vi "butterworth_waveform_filter.vi"(2 "high cutoff freq":dbl=10.0 format="%#_13g", 3 "low cutoff freq":dbl=0.05 format="%#_13g", 4 "input":waveform(dbl)(graph)) -> (1 "filtered":waveform(dbl)(graph))   [LabVIEW 2017]
uses:
  <vilib>/Analysis/3filter.llb/Filter Passband Type.ctl
  <vilib>/Analysis/3filter.llb/Butterworth Filter (DBL).vi
  <vilib>/Analysis/NI_AALBase.lvlib
panel:
  in  "order":i32=5
  out "original":waveform(dbl)(graph)
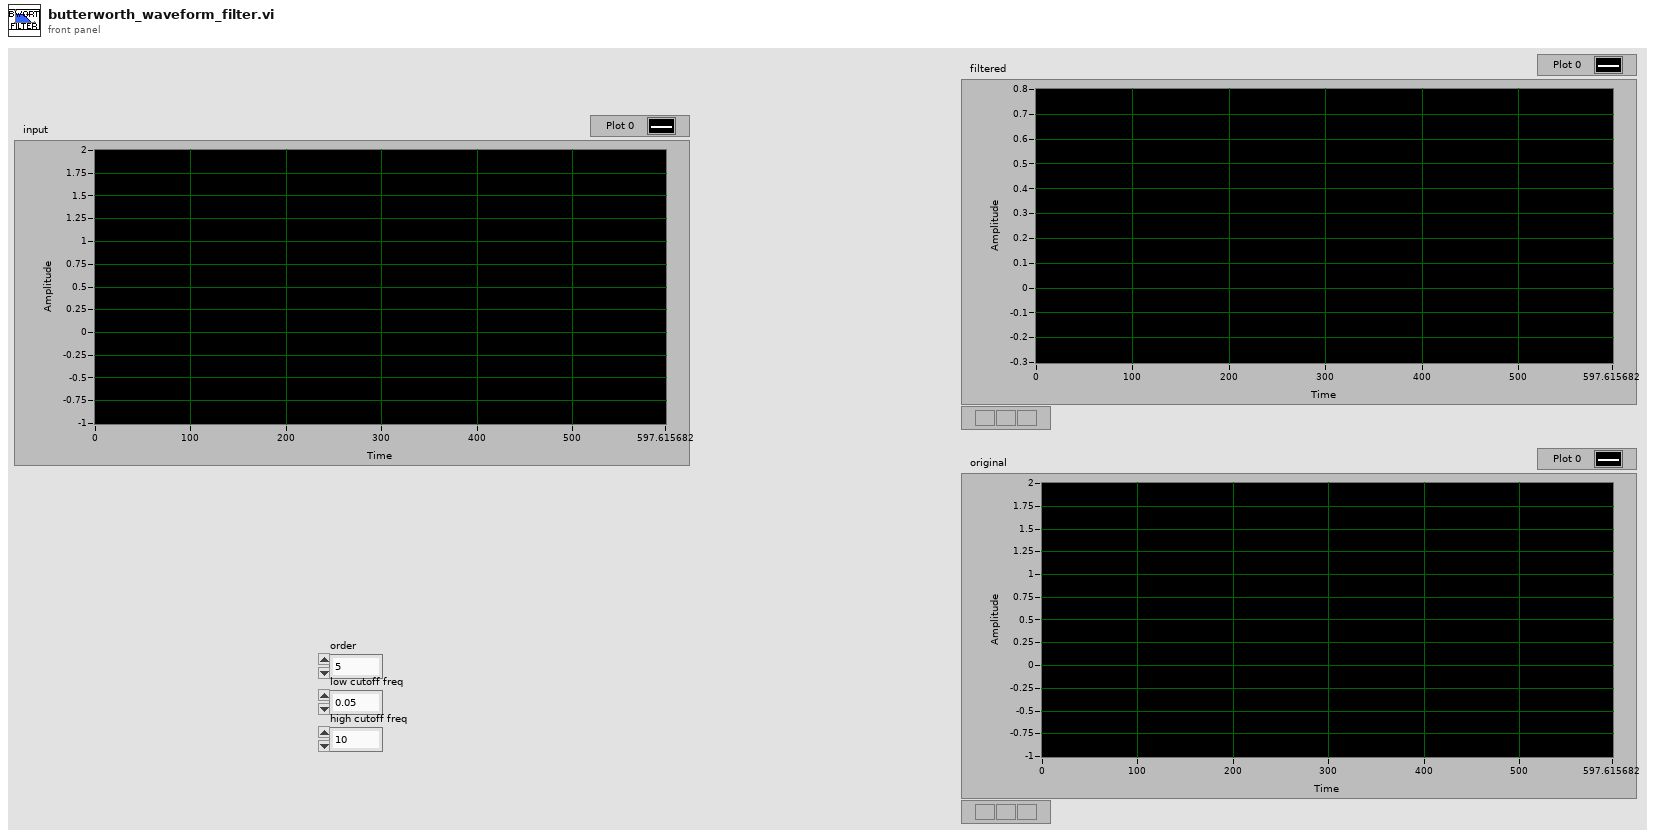
[diagram p1: front panel]
types:
  T1 = typedef "NI_AALBase.lvlib/Filter Passband Type.ctl" = enum32{"Lowpass", "Highpass", "Bandpass", "Bandstop"}
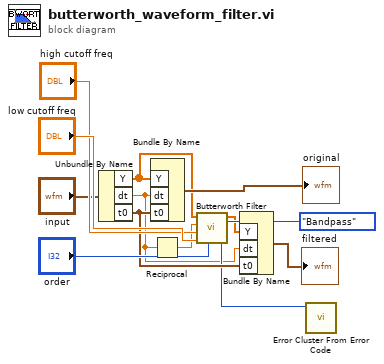
[diagram p0: block diagram]
diagram:
  n1 = Unbundle By Name("input") -> ("Y"=w6:dbl[], "dt"=w2:dbl, "t0"=w5:timestamp)
  n2 = Bundle By Name("Y"=w6, "dt"=w2, "t0"=w5) -> (→"original":waveform(dbl))  [unwired: 1 in]
  n3 = Reciprocal(x=w2) -> (1/x=w1:dbl)
  n4 = call-poly <vilib>:"Butterworth Filter.vi"("order"="order", "filter type"=Filter_Passband_Type."Bandpass", "low cutoff freq: fl"="low cutoff freq", "high cutoff freq: fh"="high cutoff freq", "sampling freq: fs"=w1, "X"=w6) -> ("error"=w3:i32, "Filtered X"=w10:dbl[])  [unwired: 2 in]
  n5 = Bundle By Name("Y"=w10, "dt"=w2, "t0"=w5) -> (→"filtered":waveform(dbl))  [unwired: 1 in]
  n6 = call <vilib>:"Error Cluster From Error Code.vi"("error code (0)"=w3) -> ()  [unwired: 8 in, 1 out]
